vi "freq to string (SubVI).vi"(11 "Frequency(Hz)":dbl(knob) min=0.0 max=200000.0 scale=500.0..1500000.0) -> (3 "string":string)   [LabVIEW 2018, in "uno3.lvlib"]
uses:
  uno3.lvlib
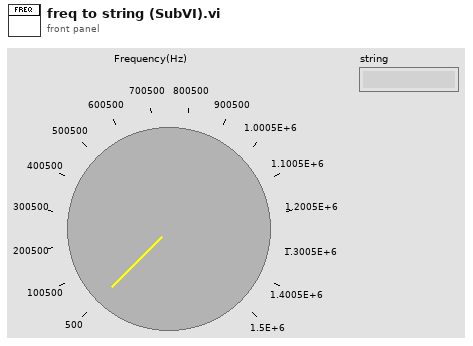
[diagram p1: front panel]
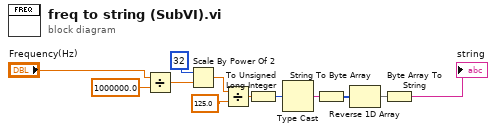
[diagram p0: block diagram]
diagram:
  n1 = Divide(x="Frequency(Hz)", y=1000000.0) -> (x/y=w7:dbl)
  n2 = Scale By Power Of 2(n=i16 32, x=w7) -> (x*2^n=w10:dbl)
  n3 = Divide(x=w10, y=125.0) -> (x/y=w12:dbl)
  n4 = To Unsigned Long Integer(number=w12) -> (unsigned 32bit integer=w6:u32)
  n5 = Type Cast(x=w6) -> (*(type *) &x=w3:string)  [unwired: 1 in]
  n6 = String To Byte Array(string=w3) -> (unsigned byte array=w5:u8[])
  n7 = Reverse 1D Array(array=w5) -> (reversed array=w4:u8[])
  n8 = Byte Array To String(unsigned byte array=w4) -> (string=→"string":string)
